vi "Read Class File Name.vi"(8 "error in (no error)":errorcluster, 11 "Generate From File in":refnum<class "Generate From File.lvclass">) -> (0 "error out":errorcluster, 2 "Class File Name":string, 3 "Generate From File out":refnum<class "Generate From File.lvclass">)   [LabVIEW 2011, in "Generate From File.lvclass"]
uses:
  Generate From File.lvclass
  Generate From File.lvclass/Generate From File.ctl
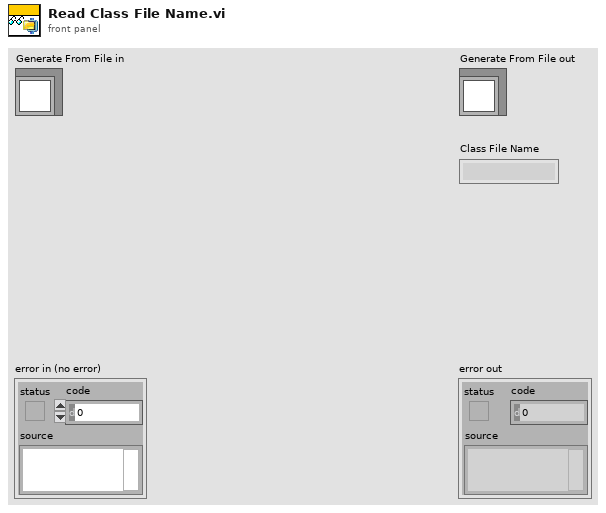
[diagram p1: front panel]
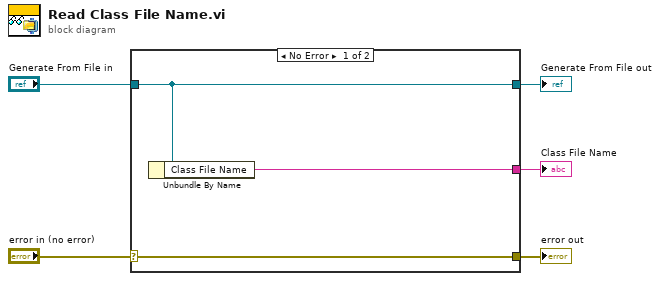
[diagram p0: block diagram]
diagram:
  n1 = case shown="No Error" "error in (no error)" {
    selector: "error in (no error)" -> [w8 w9]
    tunnel: [w8 w9] -> w4
    tunnel: [w7 w10] -> w2
    tunnel: "Generate From File in" -> [w7 w10]
    tunnel: [w6 _] -> w1
    frame No Error {
      n2 = Unbundle By Name(w7) -> ("Class File Name"=w6:string)
    }
    frame Error {
    }
  }
  "error out" <- w4
  "Generate From File out" <- w2
  "Class File Name" <- w1
